vi "autocorrelate_waveforms.vi"(9 "Y waveform":waveform(dbl), 11 "X waveform":waveform(dbl)) -> (3 "Rxx":dbl[][](array[numeric]))   [LabVIEW 2017]
uses:
  <vilib>/Analysis/2dsp.llb/2D Auto Correlation (DBL).vi
  <vilib>/Analysis/NI_AALPro.lvlib
panel:
  out "Y":dbl[](array[numeric])
  out "X":dbl[](array[numeric])
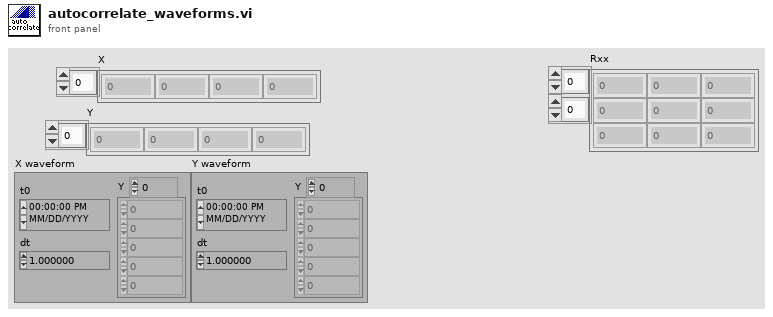
[diagram p1: front panel]
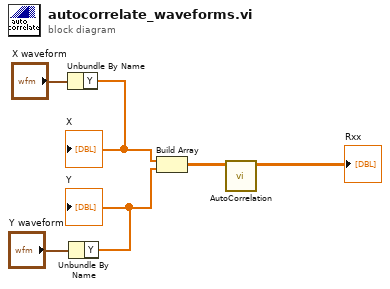
[diagram p0: block diagram]
diagram:
  n1 = Unbundle By Name("X waveform") -> ("Y"=w4:dbl[])
  "X" <- w4
  n2 = Unbundle By Name("Y waveform") -> ("Y"=w3:dbl[])
  "Y" <- w3
  n3 = Build Array(w4, w3) -> (w6:dbl[][])
  n4 = call-poly <vilib>:"AutoCorrelation.vi"("X"=w6) -> ("Rxx"=→"Rxx":dbl[][])  [unwired: 9 in, 1 out]
